vi "course.vi"(0 "x1":dbl, 5 "y 1":dbl, 7 "x2":dbl, 9 "y 2":dbl, 11 "picture":picture, 12 "color(black)":u32(colorbox)) -> (6 "new picture":picture)   [LabVIEW 2016]
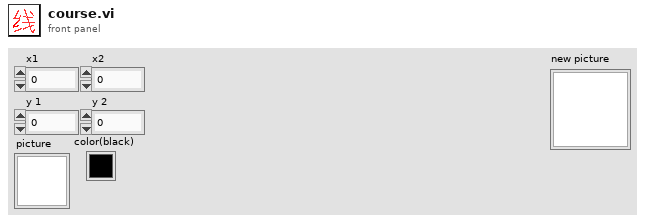
[diagram p1: front panel]
types:
  T1 = cluster{"Width":u16, "Style":enum32{"Solid", "Dash", "Dot", "DashDot", "DashDotDot"}}
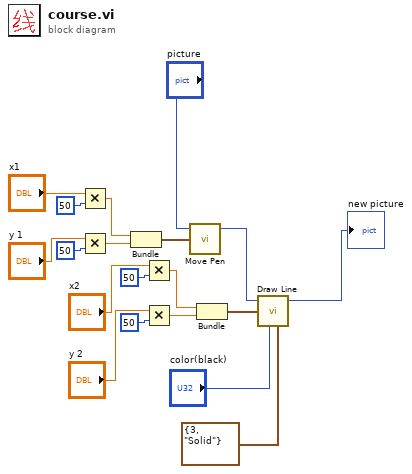
[diagram p0: block diagram]
diagram:
  n1 = Multiply(x="x1", y=50) -> (x*y=w3:dbl)
  n2 = Multiply(x="y 1", y=50) -> (x*y=w2:dbl)
  n3 = Bundle(w3, w2) -> (w14:cluster{dbl, dbl})  [unwired: 1 in]
  n4 = Multiply(x="x2", y=50) -> (x*y=w4:dbl)
  n5 = Multiply(x="y 2", y=50) -> (x*y=w1:dbl)
  n6 = call <vilib>:"Move Pen.vi"("new position"=w14, "picture"="picture") -> ("new picture"=w12:picture)  [unwired: 3 in]
  n7 = Bundle(w4, w1) -> (w18:cluster{dbl, dbl})  [unwired: 1 in]
  n8 = call <vilib>:"Draw Line.vi"("picture"=w12, "end point"=w18, "color(black)"="color(black)", "pen"=T1 {"Width"=3, "Style"=enum."Solid"}) -> ("new picture"=→"new picture":picture)  [unwired: 5 in]
